vi "APDM Get Device Data.vi"(5 "APDM Record Constant":T1, 6 "Device SN":dbl, 7 "APDM Context ID":u32) -> (2 "return type":u32, 3 "Record":T1)   [LabVIEW 2019]
uses:
  Controls/APDM Record.ctl
  Lee Lab/CP FES Walking 2018/Code/Working/LabVIEW/apdm.dll
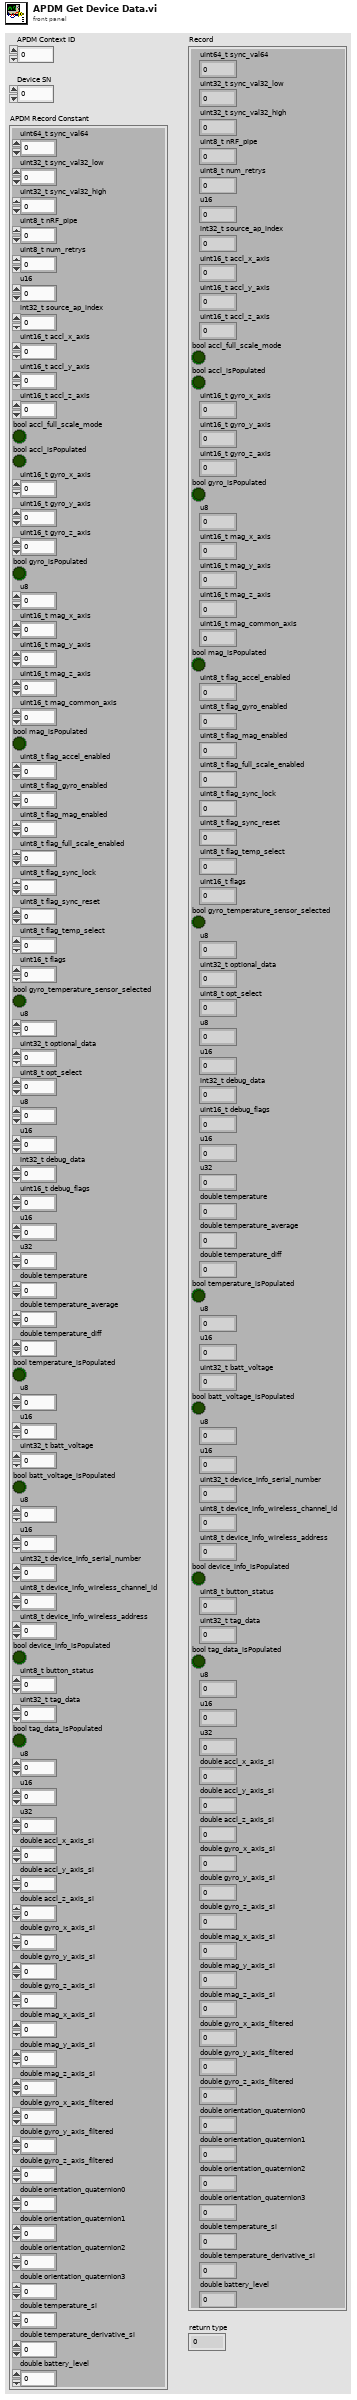
[diagram p1: front panel]
types:
  T1 = typedef "APDM Record.ctl" = cluster{"uint64_t sync_val64":u64, "uint32_t sync_val32_low":u32, "uint32_t sync_val32_high":u32, "uint8_t nRF_pipe":u8, "uint8_t num_retrys":u8, "u16":u16, "int32_t source_ap_index":i32, "uint16_t accl_x_axis":u16, "uint16_t accl_y_axis":u16, "uint16_t accl_z_axis":u16, "bool accl_full_scale_mode":bool, "bool accl_isPopulated":bool, "uint16_t gyro_x_axis":u16, "uint16_t gyro_y_axis":u16, "uint16_t gyro_z_axis":u16, "bool gyro_isPopulated":bool, "u8":u8, "uint16_t mag_x_axis":u16, "uint16_t mag_y_axis":u16, "uint16_t mag_z_axis":u16, "uint16_t mag_common_axis":u16, "bool mag_isPopulated":bool, "uint8_t flag_accel_enabled":u8, "uint8_t flag_gyro_enabled":u8, "uint8_t flag_mag_enabled":u8, "uint8_t flag_full_scale_enabled":u8, "uint8_t flag_sync_lock":u8, "uint8_t flag_sync_reset":u8, "uint8_t flag_temp_select":u8, "uint16_t flags":u16, "bool gyro_temperature_sensor_selected":bool, "u8":u8, "uint32_t optional_data":u32, "uint8_t opt_select":u8, "u8":u8, "u16":u16, "int32_t debug_data":i32, "uint16_t debug_flags":u16, "u16":u16, "u32":u32, "double temperature":dbl, "double temperature_average":dbl, "double temperature_diff":dbl, "bool temperature_isPopulated":bool, "u8":u8, "u16":u16, "uint32_t batt_voltage":u32, "bool batt_voltage_isPopulated":bool, "u8":u8, "u16":u16, "uint32_t device_info_serial_number":u32, "uint8_t device_info_wireless_channel_id":u8, "uint8_t device_info_wireless_address":u8, "bool device_info_isPopulated":bool, "uint8_t button_status":u8, "uint32_t tag_data":u32, "bool tag_data_isPopulated":bool, "u8":u8, "u16":u16, "u32":u32, "double accl_x_axis_si":dbl, "double accl_y_axis_si":dbl, "double accl_z_axis_si":dbl, "double gyro_x_axis_si":dbl, "double gyro_y_axis_si":dbl, "double gyro_z_axis_si":dbl, "double mag_x_axis_si":dbl, "double mag_y_axis_si":dbl, "double mag_z_axis_si":dbl, "double gyro_x_axis_filtered":dbl, "double gyro_y_axis_filtered":dbl, "double gyro_z_axis_filtered":dbl, "double orientation_quaternion0":dbl, "double orientation_quaternion1":dbl, "double orientation_quaternion2":dbl, "double orientation_quaternion3":dbl, "double temperature_si":dbl, "double temperature_derivative_si":dbl, "double battery_level":dbl}
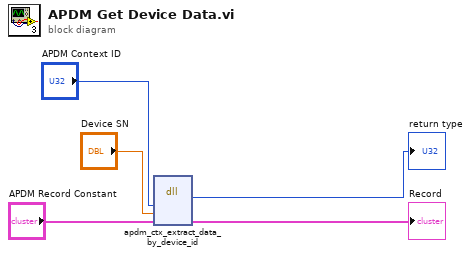
[diagram p0: block diagram]
diagram:
  n1 = dll-call lib="C:/Users/jfalesi/Dropbox/Lee Lab/CP FES Walking 2018/Code/Working/LabVIEW/apdm.dll" fn="apdm_ctx_extract_data_by_device_id"("context"="APDM Context ID", "dev ID"="Device SN", "Record"="APDM Record Constant") -> ("return type"=→"return type":u32, "Record"=→"Record":T1)  [unwired: 5 in, 2 out]
